vi "Shutdown.vi"(8 "Error In":errorcluster, 11 "SSH":refnum<class "SSH.lvclass">) -> (0 "Error Out":errorcluster)   [LabVIEW 2021, in "Field_RnD_Services_LIBSSH2_Toolkit.lvlib" / "SSH.lvclass"]
doc: "Cleanly and safely shutdowns the underlying libssh2lv shared library. This must be called, or executed, after all other VIs within this toolkit are completed. Once this is called, no other VIs from this toolkit should be called, or executed. This frees all internal memory used by the libssh2lv shared library. A segmentation fault will occur if toolkit VIs are executed after this VI is executed."
uses:
  SSH.lvclass
  SSH.lvclass/SSH.ctl
  Field_RnD_Services_LIBSSH2_Toolkit.lvlib
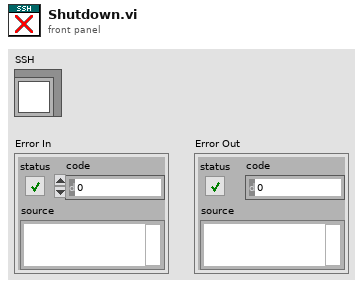
[diagram p1: front panel]
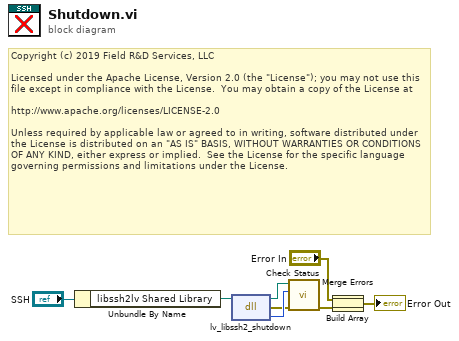
[diagram p0: block diagram]
diagram:
  # "Copyright (c) 2019 Field R&D Services, LLC\n\nLicensed under the Apache License, Version 2.0 (the \"License\"); you may not use this file except in compliance with the License.  You may obtain a copy of the License at\n\nhttp://www.apache.org/licenses/LICENSE-2.0\n\nUnless required by applicable law or agreed to in writing, software distributed under the License is distributed on an \"AS IS\" BASIS, WITHOUT WARRANTIES OR CONDITIONS OF ANY KIND, either express or implied.  See the License for the specific language governing permissions and limitations under the License."
  n1 = Unbundle By Name("SSH") -> ("libssh2lv Shared Library"=w3:path)
  n2 = dll-call lib="libssh2lv.*" fn="lv_libssh2_shutdown"(path in=w3) -> (path out=w7:path, error out=w5:errorcluster, "return type"=w6:i32)  [unwired: 2 in]
  n3 = call "Check Status.vi"("Error In"=w5, "Status"=w6, "libssh2lv Shared Library In"=w7) -> ("Error Out"=w2:errorcluster)  [unwired: 7 in, 1 out]
  n4 = Build Array("Error In", w2) -> (w1:errorcluster[])
  n5 = Merge Errors(w1) -> (→"Error Out":errorcluster)
